vi "Length offset.vi"(11 "Folder Path":path) -> (2 "Length":i32, 3 "Offset":i32)   [LabVIEW 2016]
uses:
  Number of Events Global.vi
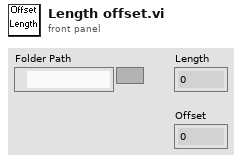
[diagram p1: front panel]
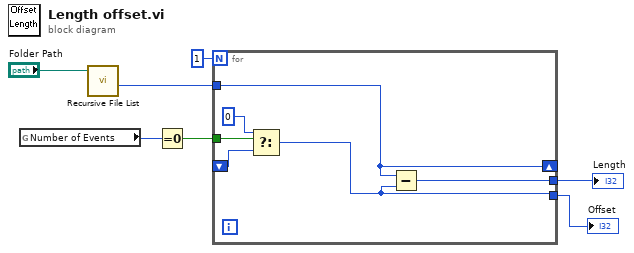
[diagram p0: block diagram]
diagram:
  n1 = global read "Number of Events Global.vi" "Number of Events"() -> (w2:i32)
  n2 = call <vilib>:"Recursive File List.vi"("Folder Path"="Folder Path") -> ("Number of Files"=w4:i32)  [unwired: 7 in, 3 out]
  n3 = Equal To 0?(x=w2) -> (x = 0?=w1:bool)
  n4 = for {
    N: 1 -> [_]
    tunnel: w4 -> [w13]
    shift-right: [w13] -> _
    shift-left: _ -> [w9]
    tunnel: [w10] -> w6
    tunnel: [w12] -> w5
    tunnel: w1 -> [w11]
    n5 = Select(t=0, s=w11, f=w9) -> (s? t:f=w10:i32)
    n6 = Subtract(x=w13, y=w10) -> (x-y=w12:i32)
  }
  "Offset" <- w6
  "Length" <- w5
